vi "Get Boolean.vi"(1 "Name":string) -> (0 "Value":bool)   [LabVIEW 2017, in "Apple script.lvlib"]
doc: "Used to retrieve boolean values for use in \"until\" subcommands."
uses:
  Apple script.lvlib
  Support Code/Support Code.lvlib
panel:
  in  "Test Boolean":bool
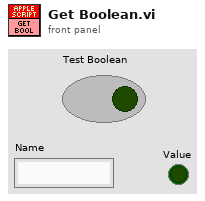
[diagram p1: front panel]
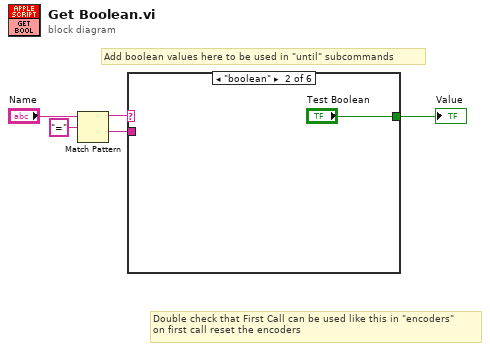
[diagram p0: block diagram]
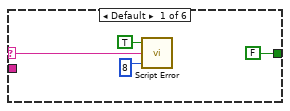
[diagram p2: hidden frame]
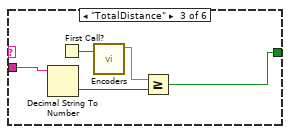
[diagram p3: hidden frame]
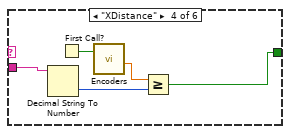
[diagram p4: hidden frame]
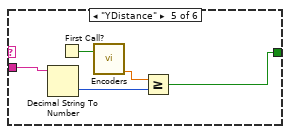
[diagram p5: hidden frame]
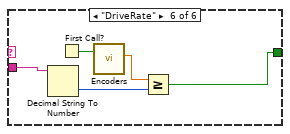
[diagram p6: hidden frame]
diagram:
  # "Double check that First Call can be used like this in \"encoders\"\non first call reset the encoders"
  # "Add boolean values here to be used in \"until\" subcommands"
  n1 = Match Pattern(string="Name", regular expression="=") -> (before substring=w3:string, after substring=w1:string)  [unwired: 1 in, 2 out]
  n2 = case shown="\"boolean\"" w3 {
    selector: w3 -> [w6 _ _ _ _ _]
    tunnel: [FALSE "Test Boolean" w12 w18 w23 w28] -> w5
    tunnel: w1 -> [_ _ w13 w19 w24 w29]
    frame Default {
      n3 = call "Script Error.vi"("Error?"=TRUE, "Error Details"=w6, "Error Code"=8) -> ()  [unwired: 2 in, 1 out]
    }
    frame "boolean" {
    }
    frame "TotalDistance" {
      n4 = Decimal String To Number(string=w13) -> (number=w11:i32)  [unwired: 2 in, 1 out]
      n5 = First Call?() -> (First Call?: T/F=w15:bool)
      n6 = call "Encoders.vi"("Reset Encoders?"=w15) -> ("Total Distance"=w14:dbl)  [unwired: 2 in, 3 out]
      n7 = Greater Or Equal?(x=w14, y=w11) -> (x >= y?=w12:bool)
    }
    frame "XDistance" {
      n8 = Decimal String To Number(string=w19) -> (number=w17:i32)  [unwired: 2 in, 1 out]
      n9 = First Call?() -> (First Call?: T/F=w20:bool)
      n10 = call "Encoders.vi"("Reset Encoders?"=w20) -> ("X Distance"=w16:dbl)  [unwired: 2 in, 3 out]
      n11 = Greater Or Equal?(x=w16, y=w17) -> (x >= y?=w18:bool)
    }
    frame "YDistance" {
      n12 = Decimal String To Number(string=w24) -> (number=w22:i32)  [unwired: 2 in, 1 out]
      n13 = First Call?() -> (First Call?: T/F=w25:bool)
      n14 = call "Encoders.vi"("Reset Encoders?"=w25) -> ("Y Distance"=w21:dbl)  [unwired: 2 in, 3 out]
      n15 = Greater Or Equal?(x=w21, y=w22) -> (x >= y?=w23:bool)
    }
    frame "DriveRate" {
      n16 = Decimal String To Number(string=w29) -> (number=w27:i32)  [unwired: 2 in, 1 out]
      n17 = First Call?() -> (First Call?: T/F=w30:bool)
      n18 = call "Encoders.vi"("Reset Encoders?"=w30) -> ("Avg Rate"=w26:dbl)  [unwired: 2 in, 3 out]
      n19 = Greater Or Equal?(x=w26, y=w27) -> (x >= y?=w28:bool)
    }
  }
  "Value" <- w5
